vi "Cleanup.vi"(8 "error in (no error)":errorcluster, 11 "Square Field Panel in":refnum<class "Square Field Panel.lvclass">) -> (0 "error out":errorcluster)   [LabVIEW 2020, in "SB App.lvlib" / "Square Field Panel.lvclass"]
uses:
  Square Field Panel.lvclass
  Square Field Panel.lvclass/Square Field Panel.ctl
  <vilib>/IlluminatedG/IG OOPanel/OOPanel/Panel/Panel.lvclass
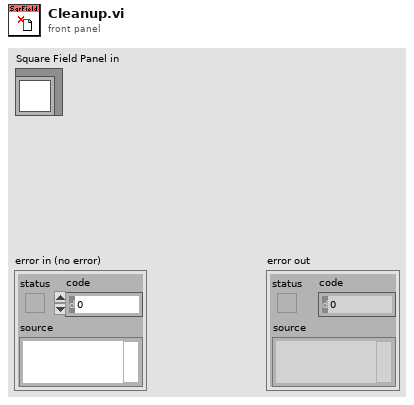
[diagram p1: front panel]
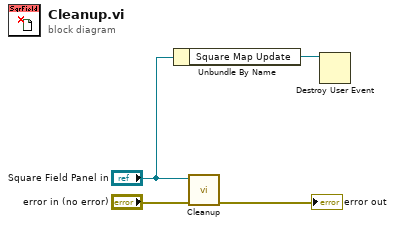
[diagram p0: block diagram]
diagram:
  n1 = Unbundle By Name("Square Field Panel in") -> ("Square Map Update"=w1:refnum<user-event>)
  n2 = call-parent "Cleanup.vi"("error in (no error)"="error in (no error)", "Panel in"="Square Field Panel in") -> ("error out"=→"error out":errorcluster)  [unwired: 9 in]
  n3 = Destroy User Event(user event=w1) -> ()  [unwired: 1 in, 1 out]
